vi "Init.vi"(8 "error in (no error)":errorcluster, 10 "Muxes":cluster{"Mux Route":i32[]}[](array[cluster])) -> (0 "error out":errorcluster, 3 "MuxRoute Value out":refnum<class "MuxRoute Value.lvclass">)   [LabVIEW 2022 SP3, in "VideoMux.lvlib" / "MuxRoute Value.lvclass"]
uses:
  MuxRoute Value.lvclass
  MuxRoute Value.lvclass/MuxRoute Value.ctl
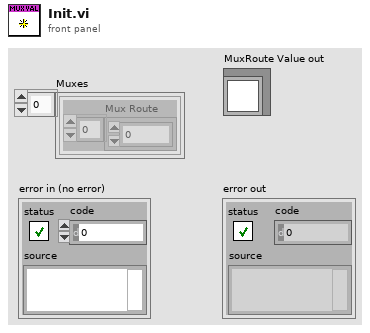
[diagram p1: front panel]
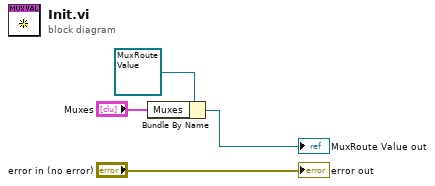
[diagram p0: block diagram]
diagram:
  n1 = Bundle By Name(cluster=refnum<class "MuxRoute Value.lvclass"> refnum ("MuxRoute Value in"), "Muxes"="Muxes") -> (→"MuxRoute Value out":refnum<class "MuxRoute Value.lvclass">)
  "error out" <- "error in (no error)"
